vi "Read Always Repeat First Node.vi"(8 "error in (no error)":errorcluster, 11 "Parallel_Interleaved in":refnum<class "bt_Parallel_Interleaved.lvclass">) -> (0 "error out":errorcluster, 2 "Always Repeat First Node":bool, 3 "Parallel_Interleaved out":refnum<class "bt_Parallel_Interleaved.lvclass">)   [LabVIEW 2021, in "BT.lvlib" / "bt_Parallel_Interleaved.lvclass"]
uses:
  bt_Parallel_Interleaved.lvclass
  bt_Parallel_Interleaved.lvclass/bt_Parallel_Interleaved.ctl
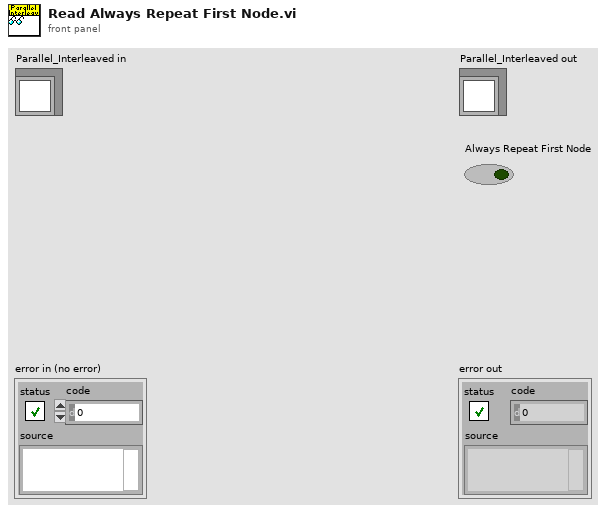
[diagram p1: front panel]
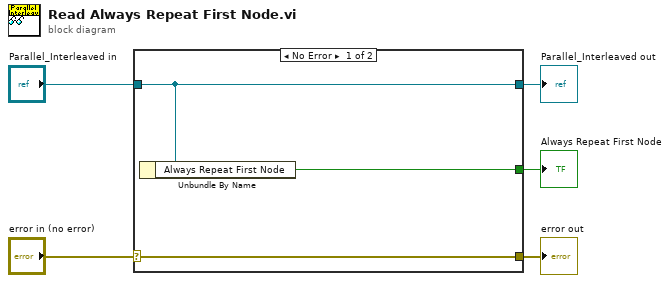
[diagram p0: block diagram]
diagram:
  n1 = case shown="No Error" "error in (no error)" {
    selector: "error in (no error)" -> [w8 w9]
    tunnel: [w8 w9] -> w4
    tunnel: [w7 w10] -> w2
    tunnel: "Parallel_Interleaved in" -> [w7 w10]
    tunnel: [w6 _] -> w1
    frame No Error {
      n2 = Unbundle By Name(w7) -> ("Always Repeat First Node"=w6:bool)
    }
    frame Error {
    }
  }
  "error out" <- w4
  "Parallel_Interleaved out" <- w2
  "Always Repeat First Node" <- w1
